vi "Read target.vi"(8 "error in (no error)":errorcluster, 11 "TargetConfiguration in":refnum<class "TargetConfiguration.lvclass">) -> (0 "error out":errorcluster, 2 "Target.lvclass":refnum<class "Target.lvclass">, 3 "TargetConfiguration out":refnum<class "TargetConfiguration.lvclass">)   [LabVIEW 2014, in "TCSDataDefinitions.lvlib" / "TCSCommand.lvlib" / "TargetConfiguration.lvlib" / "TargetConfiguration.lvclass"]
uses:
  TargetConfiguration.lvclass
  Target/Target/Target.lvclass
  TargetConfiguration.lvclass/TargetConfiguration.ctl
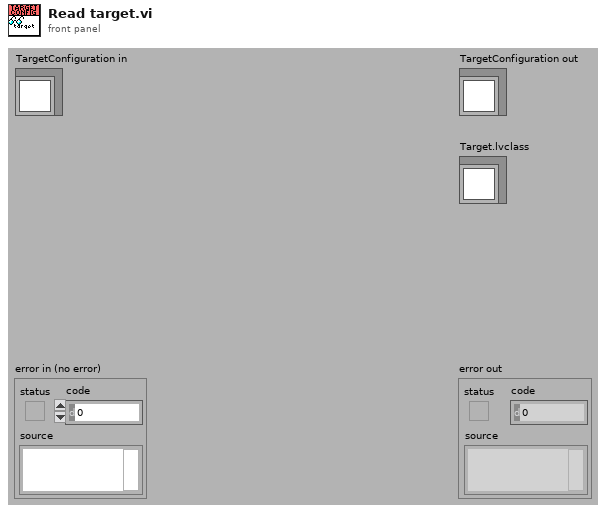
[diagram p1: front panel]
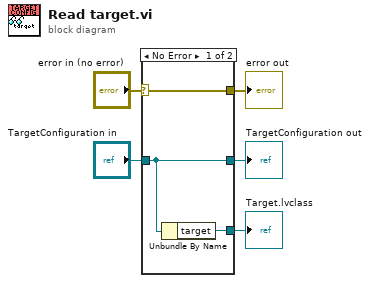
[diagram p0: block diagram]
diagram:
  n1 = case shown="No Error" "error in (no error)" {
    selector: "error in (no error)" -> [w8 w9]
    tunnel: [w8 w9] -> w4
    tunnel: [w7 w10] -> w2
    tunnel: "TargetConfiguration in" -> [w7 w10]
    tunnel: [w6 _] -> w1
    frame No Error {
      n2 = Unbundle By Name(w7) -> ("target"=w6:refnum<class "Target.lvclass">)
    }
    frame Error {
    }
  }
  "error out" <- w4
  "TargetConfiguration out" <- w2
  "Target.lvclass" <- w1
